vi "writ data to plc.vi"(7 "action":T1(ring)=enum."internal relay(M)", 8 "Start address":i32, 10 "M":bool[](array[boolean]), 11 "D":dbl[](array[numeric])=[1234.0, 5678.0, 9876.0]) -> (3 "Out":string)   [LabVIEW 2015]
panel:
  out "String":string
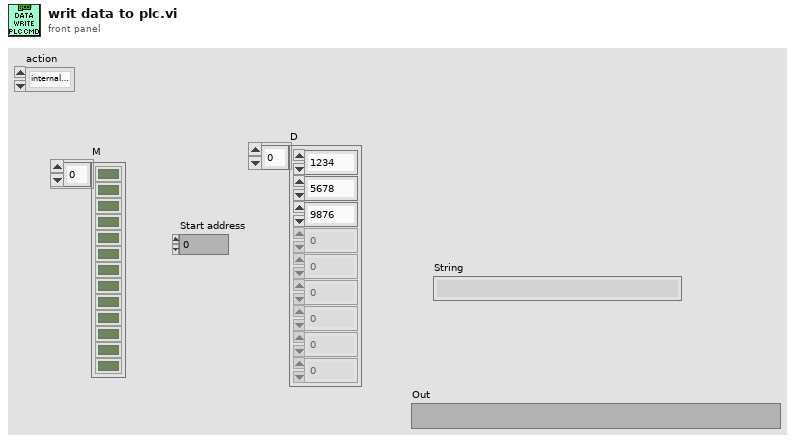
[diagram p1: front panel]
types:
  T1 = enum16{"Input(X)", "Output(Y)", "internal relay(M)", "Data Register(D)"}
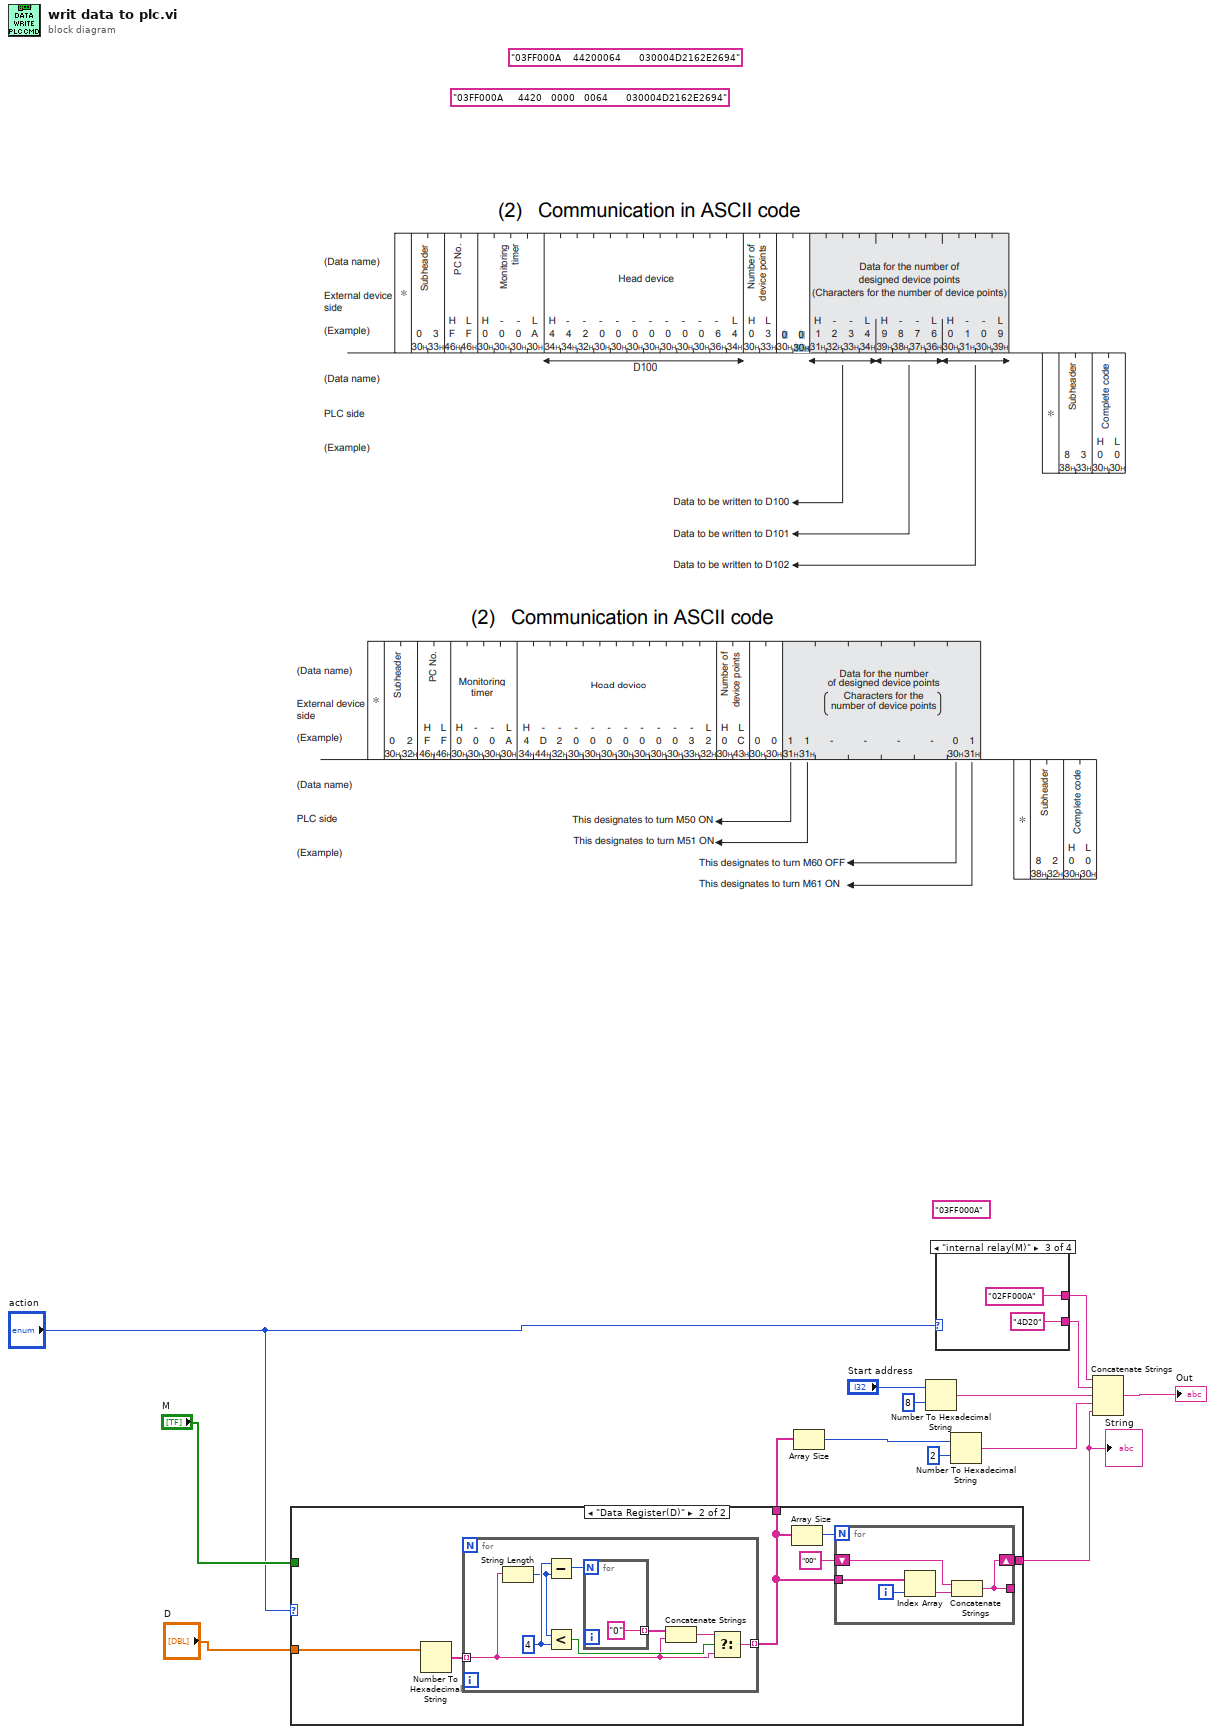
[diagram p0: block diagram]
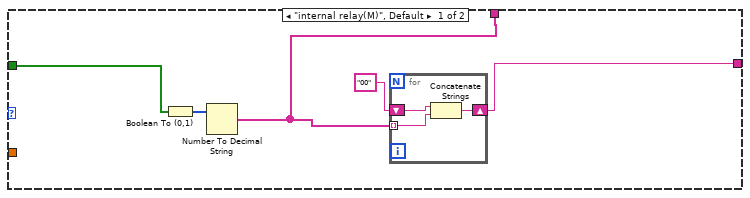
[diagram p2: hidden frame]
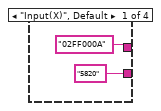
[diagram p3: hidden frame]
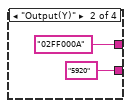
[diagram p4: hidden frame]
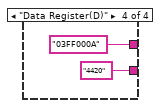
[diagram p5: hidden frame]
diagram:
  (unwired) "03FF000A     4420   0000   0064      030004D2162E2694" ("Out 2")
  (unwired) "03FF000A    44200064      030004D2162E2694" ("Out 2")
  (unwired) "03FF000A" ("Command")
  n1 = case shown="\"Data Register(D)\"" "action" {
    tunnel: [w16 w26] -> w14
    tunnel: [w17 w24] -> w8
    tunnel: "M" -> [w15 _]
    tunnel: "D" -> [_ w23]
    frame "internal relay(M)", Default {
      n2 = Boolean To (0,1)(Boolean=w15) -> (0, 1=w18:i16[])
      n3 = Number To Decimal String(number=w18) -> (decimal integer string=w16:string[])  [unwired: 1 in]
      n4 = for {
        tunnel: w16 -> [w22] mode=indexing
        shift-right: [w20] -> w17
        shift-left: "00" -> [w21]
        n5 = Concatenate Strings(w21, w22) -> (w20:string)
      }
    }
    frame "Data Register(D)" {
      n6 = Number To Hexadecimal String(2:w23) -> (0:w25:string[])  [unwired: 1 in]
      n7 = for {
        tunnel: w25 -> [w31] mode=indexing
        tunnel: [w29] -> w26 mode=indexing
        w35 = 4 ("y")
        n8 = String Length(string=w31) -> (length=w34:i32)
        n9 = Subtract(x=w35, y=w34) -> (x-y=w33:i32)
        n10 = Less?(x=w34, y=w35) -> (x < y?=w36:bool)
        n11 = for {
          N: w33 -> [_]
          tunnel: ["0"] -> w32 mode=indexing
        }
        n12 = Concatenate Strings(w32, w31) -> (w30:string)
        n13 = Select(t=w30, s=w36, f=w31) -> (s? t:f=w29:string)
      }
      n14 = Array Size(array=w26) -> (size(s)=w27:i32)
      n15 = for {
        N: w27 -> [_]
        shift-right: [w40] -> w24
        shift-left: "00" -> [w39]
        tunnel: [w40] -> _
        tunnel: w26 -> [w38]
        i -> [w42]
        n16 = Index Array(array=w38, index=w42) -> (element=w41:string)
        n17 = Concatenate Strings(w39, w41) -> (w40:string)
      }
    }
  }
  "String" <- w8
  n18 = Array Size(array=w14) -> (size(s)=w6:i32)
  n19 = Number To Hexadecimal String(1:i16 8 ("width (-)"), 2:"Start address") -> (0:w11:string)
  n20 = case shown="\"internal relay(M)\"" "action" {
    tunnel: ["5820" ("Command") "5920" ("Command") "4D20" ("Command") "4420" ("Command")] -> w9
    tunnel: ["02FF000A" ("Command") "02FF000A" ("Command") "02FF000A" ("Command") "03FF000A" ("Command")] -> w4
    frame "Input(X)", Default {
    }
    frame "Output(Y)" {
    }
    frame "internal relay(M)" {
    }
    frame "Data Register(D)" {
    }
  }
  n21 = Number To Hexadecimal String(1:i16 2 ("width (-)"), 2:w6) -> (0:w5:string)
  n22 = Concatenate Strings(w4, w9, w11, w5, w8) -> (→"Out":string)
